vi "Device tester (speaker).vi"() -> ()   [LabVIEW 2011]
uses:
  Device/Typedefs/Speaker.ctl
  Rack/Typedefs/OutputRequest refnum.ctl
  Rack/Typedefs/OutputRequest.ctl
  Rack/Typedefs/InputData cluster.ctl
  Rack/Methods/Port drivers/DigitalInput-DataCluster.ctl
  Rack/Methods/Rack-Init.vi
  Device/Methods/Speaker-Init.vi
  Rack/Methods/Rack-Config.vi
  Rack/Methods/Rack-Start.vi
  Rack/Methods/Rack-Stop.vi
  Device/Methods/Speaker-Play.vi
  Device/Methods/Speaker-PlaySequence.vi
panel:
  in  "Sine sequence":T1(array[cluster])
  in  "Play sequence":bool
  in  "Amplitude (V)":dbl=0.1
  in  "Duration (ms)":dbl=100.0
  in  "Frequency (Hz)":dbl=1000.0
  in  "Speaker":T2={"Settings"={"Portname"="BNC_Panel.ao0", "Index"=0, "Timestamp portname"="BNC_Panel.P0.0"}, "OutputRequest event ref"=refnum, "InputData reference"=refnum}
  in  "stop":bool
  in  "Play":bool
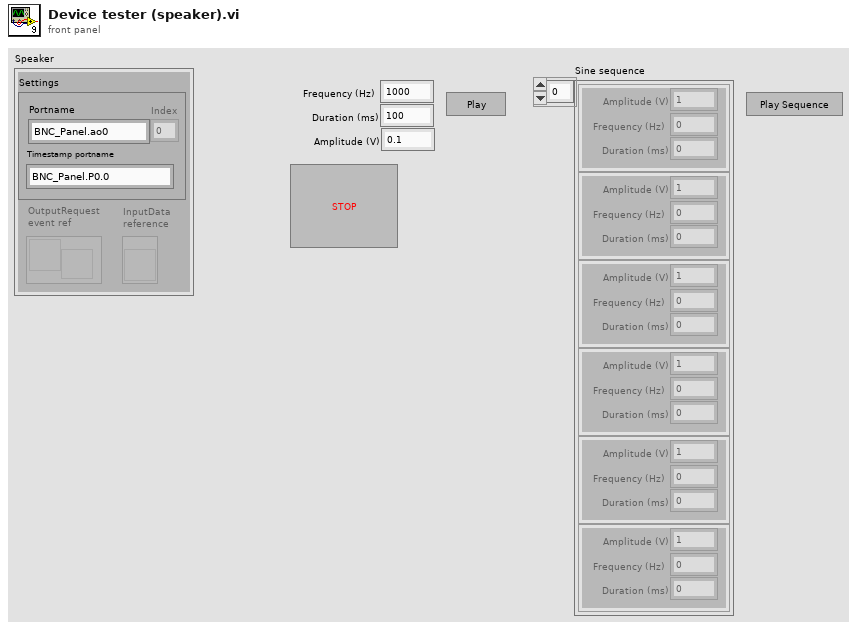
[diagram p1: front panel]
types:
  T1 = cluster{"Frequency (Hz)":dbl, "Duration (ms)":dbl, "Amplitude (V)":dbl}[]
  T2 = typedef "Speaker.ctl" = cluster{"Settings":cluster{"Portname":string, "Index":i32, "Timestamp portname":string}, "OutputRequest event ref":T3, "InputData reference":refnum<vi>}
  T3 = typedef "OutputRequest refnum.ctl" = refnum<user-event>
  T4 = typedef "Rack driver configuration cluster.ctl" = cluster{"DigitalInput":T5, "DigitalOutput":T6, "FileOutput":T7, "AnalogOutput":T8, "DataSocketOutput":T9}
  T5 = typedef "DigitalInput-Configuration.ctl" = cluster{"Lines":tag[], "Refresh period (ms)":u32}
  T6 = typedef "DigitalOutput-Configuration.ctl" = cluster{"Output Lines":tag[], "DO timestamp lines":tag[], "Timestamp lines":tag[]}
  T7 = typedef "FileOutput-Configuration.ctl" = cluster{"Logfile path":path}
  T8 = typedef "AnalogOutput-Configuration.ctl" = cluster{"Output Lines":tag[], "AO timestamp lines":tag[]}
  T9 = typedef "DataSocketOutput-Configuration.ctl" = cluster{"DataSocket URL":string}
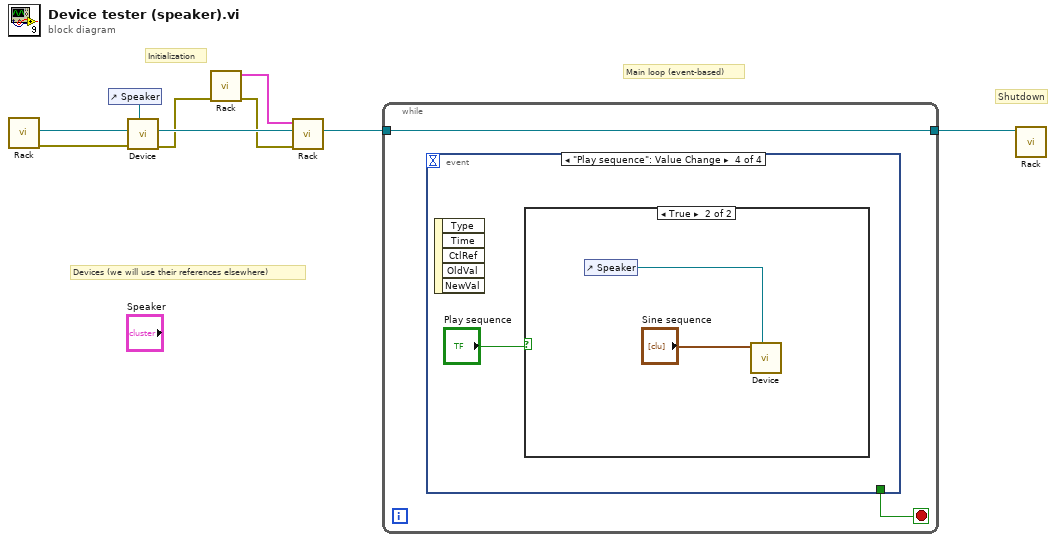
[diagram p0: block diagram]
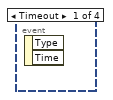
[diagram p2: hidden frame]
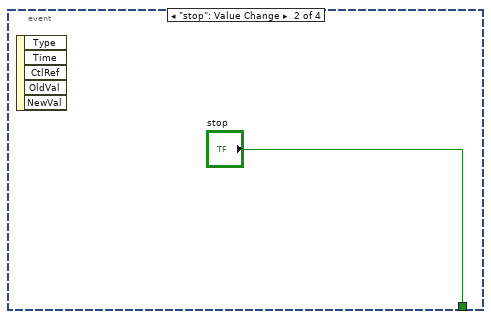
[diagram p3: hidden frame]
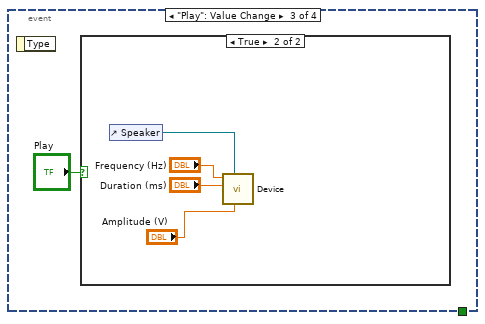
[diagram p4: hidden frame]
diagram:
  # "Main loop (event-based)"
  # "Shutdown"
  # "Initialization"
  # "Devices (we will use their references elsewhere)"
  n1 = call-poly "Rack.vi"() -> ("error out"=w3:errorcluster, "OutputRequest\nevent ref"=w7:T3)  [unwired: 10 in]
  n2 = control-ref of="Speaker"() -> (w1:refnum<vi>)
  n3 = call-poly "Device.vi"("Device reference"=w1, "error in (no error)"=w3, "OutputRequest event ref"=w7) -> ("error out"=w4:errorcluster, "OutputRequest (dup)"=w6:T3)  [unwired: 6 in, 1 out]
  n4 = call-poly "Rack.vi"("error in (no error)"=w4) -> ("error out"=w2:errorcluster, "Configuration"=w9:T4)  [unwired: 9 in]
  n5 = call-poly "Rack.vi"("error in (no error)"=w2, "OutputRequest event ref"=w6, "Configuration"=w9) -> ("OutputRequest event ref (dup)"=w5:T3)  [unwired: 7 in, 1 out]
  n6 = while {
    tunnel: w5 -> [w10]
    tunnel: [w10] -> w8
    stop <- w11 stop-if-true
    n7 = event shown="[3] \"Play sequence\": Value Change" {
      selector: _ -> [_ _ _ _]
      dyn-events: _ -> [_ _ _ _]
      timeout: _ -> [_ _ _ _]
      tunnel: [_ "stop" _ _] -> w11
      event Timeout {
        n8 = event-data() -> ()  [unwired: 1 in, 2 out]
      }
      event "stop": Value Change {
        n9 = event-data() -> ()  [unwired: 1 in, 5 out]
      }
      event "Play": Value Change {
        n10 = event-data() -> ()  [unwired: 1 in, 1 out]
        n11 = case shown="True" "Play" {
          frame False {
          }
          frame True {
            n12 = control-ref of="Speaker"() -> (w17:refnum<vi>)
            n13 = call-poly "Device.vi"("Amplitude (V)"="Amplitude (V)", "Device reference"=w17, "Duration (ms)"="Duration (ms)", "Frequency (Hz)"="Frequency (Hz)") -> ()  [unwired: 7 in, 1 out]
          }
        }
      }
      event "Play sequence": Value Change {
        n14 = event-data() -> ()  [unwired: 1 in, 5 out]
        n15 = case shown="True" "Play sequence" {
          frame False {
          }
          frame True {
            n16 = control-ref of="Speaker"() -> (w20:refnum<vi>)
            n17 = call-poly "Device.vi"("Device reference"=w20, "Sine sequence"="Sine sequence") -> ()  [unwired: 9 in, 1 out]
          }
        }
      }
    }
  }
  n18 = call-poly "Rack.vi"("OutputRequest channel"=w8) -> ()  [unwired: 10 in, 1 out]
